vi "SAOMM-FalconFixer.vi"(0 "PRAMMS VRN":refnum<visa-resource-name>="COM4", 1 "ROIYOffset":u16, 2 "ROIXOffset":u16, 3 "Binning":u16(ring) items=["1 x 1"=1, "2 x 2"=2, "4 x 4"=4, "5 x 5"=5], 7 "Signature":u32, 11 "PRAMMS Error":errorcluster, 12 "ROIWidth":u16, 13 "ROIHeight":u16) -> ()   [LabVIEW 2011]
uses:
  Polymorphics/Num2littleEndian(U16).vi
panel:
  out "appended array 2":bool[](array[boolean])
  out "DumpArray1":string[](array[string])
  out "appended array":bool[](array[boolean])
  out "Boolean":bool
  out "DumpArray2":string[](array[string])
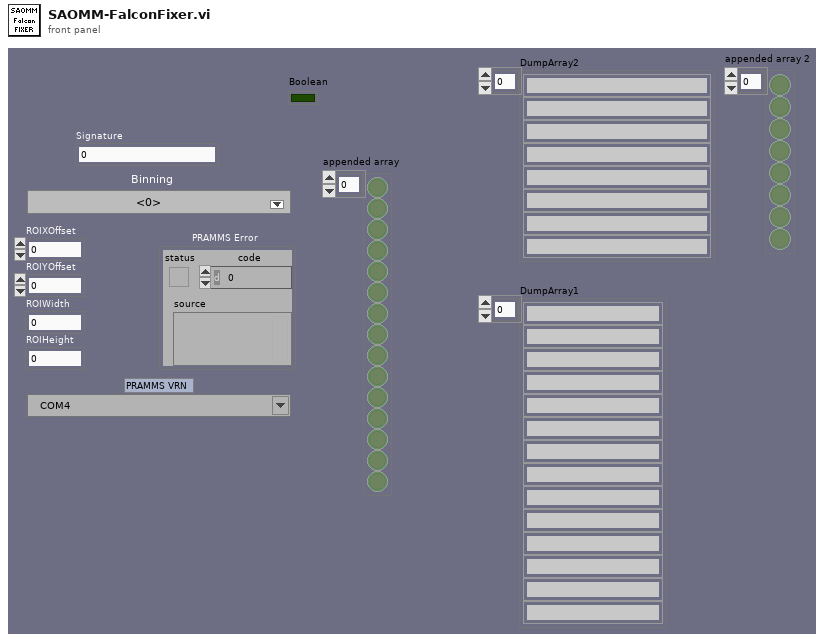
[diagram p1: front panel]
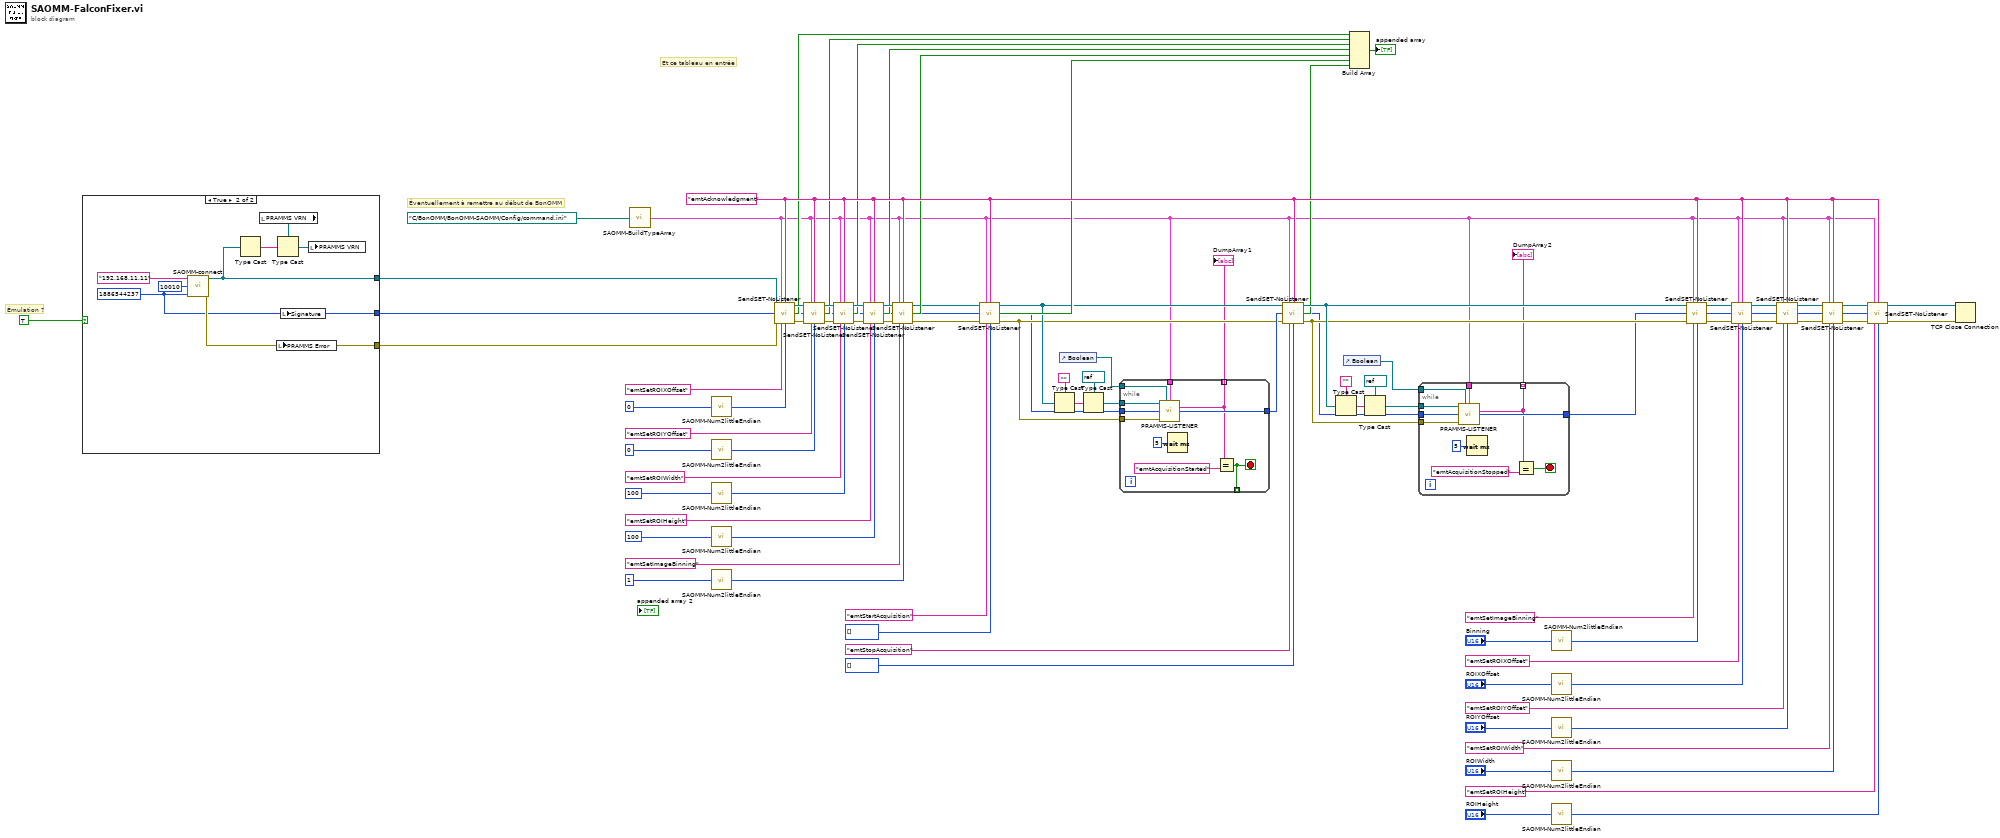
[diagram p0: block diagram]
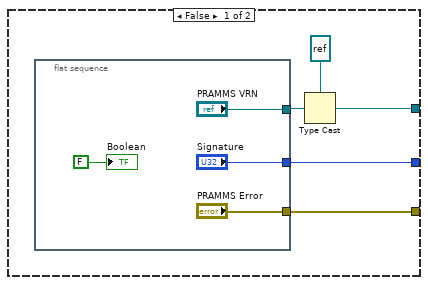
[diagram p2: hidden frame]
diagram:
  w48 = "emtAcknowledgment" ("ExpectedAnswer")
  # "Émulation ?"
  # "Et ce tableau en entrée"
  # "Éventuellement à remettre au début de BonOMM"
  n1 = case shown="True" TRUE {
    tunnel: [w92 w97] -> w69
    tunnel: [w89 w102] -> w50
    tunnel: [w88 w101] -> w3
    frame False {
      n2 = flat-sequence {
        tunnel: ["PRAMMS VRN"] -> w90
        tunnel: ["PRAMMS Error"] -> w89
        tunnel: ["Signature"] -> w88
        frame #0 {
          "Boolean" <- FALSE
        }
      }
      n3 = Type Cast(type=refnum<k5> refnum ("connection ID"), x=w90) -> (*(type *) &x=w92:refnum<k5>)
    }
    frame True {
      w101 = u32 1886544237 ("Signature")
      n4 = call "SAOMM-connect.vi"("IP"="192.168.11.11", "Port"=u16 10010, "Signature"=w101) -> ("connection ID"=w97:refnum<k5>, "Error OUT"=w102:errorcluster)  [unwired: 8 in, 3 out]
      n5 = Type Cast(x=w97) -> (*(type *) &x=w98:string)  [unwired: 1 in]
      n6 = local read "PRAMMS VRN"() -> (w100:refnum<visa-resource-name>)
      n7 = local write "PRAMMS Error"(w102) -> ()
      n8 = Type Cast(type=w100, x=w98) -> (*(type *) &x=w99:refnum<visa-resource-name>)
      n9 = local write "Signature"(w101) -> ()
      n10 = local write "PRAMMS VRN"(w99) -> ()
    }
  }
  n11 = call "SAOMM-BuildTypeArray.vi"("command.ini"=path "C:/BonOMM/BonOMM-SAOMM/Config/command.ini") -> ("CommandArray"=w9:cluster{string[], u32[]})  [unwired: 14 in]
  n12 = call-poly "SAOMM-Num2littleEndian.vi"("Number"=u16 0) -> ("LiitleEndianedData"=w63:u8[])  [unwired: 14 in]
  n13 = call-poly "SAOMM-Num2littleEndian.vi"("Number"=u16 0) -> ("LiitleEndianedData"=w62:u8[])  [unwired: 14 in]
  n14 = call-poly "SAOMM-Num2littleEndian.vi"("Number"=u16 100) -> ("LiitleEndianedData"=w61:u8[])  [unwired: 14 in]
  n15 = call-poly "SAOMM-Num2littleEndian.vi"("Number"=u16 100) -> ("LiitleEndianedData"=w60:u8[])  [unwired: 14 in]
  n16 = call-poly "SAOMM-Num2littleEndian.vi"("Number"=u16 1) -> ("LiitleEndianedData"=w56:u8[])  [unwired: 14 in]
  n17 = call "SendSET-NoListener.vi"("connection ID"=w69, "CommandArray"=w9, "ExpectedAnswer"=w48, "Signature"=w3, "Error IN"=w50, "Active SET"="emtSetROIXOffset", "Value (little endianed byte array)"=w63) -> ("connection ID (dup)"=w82:refnum<k5>, "Succes"=w25:bool, "Error OUT"=w68:errorcluster)  [unwired: 6 in]
  n18 = call "SendSET-NoListener.vi"("connection ID"=w82, "CommandArray"=w9, "ExpectedAnswer"=w48, "Signature"=w3, "Error IN"=w68, "Active SET"="emtSetROIYOffset", "Value (little endianed byte array)"=w62) -> ("connection ID (dup)"=w81:refnum<k5>, "Succes"=w24:bool, "Error OUT"=w73:errorcluster)  [unwired: 6 in]
  n19 = call "SendSET-NoListener.vi"("connection ID"=w81, "CommandArray"=w9, "ExpectedAnswer"=w48, "Signature"=w3, "Error IN"=w73, "Active SET"="emtSetROIWidth", "Value (little endianed byte array)"=w61) -> ("connection ID (dup)"=w80:refnum<k5>, "Succes"=w23:bool, "Error OUT"=w70:errorcluster)  [unwired: 6 in]
  n20 = call "SendSET-NoListener.vi"("connection ID"=w80, "CommandArray"=w9, "ExpectedAnswer"=w48, "Signature"=w3, "Error IN"=w70, "Active SET"="emtSetROIHeight", "Value (little endianed byte array)"=w60) -> ("connection ID (dup)"=w58:refnum<k5>, "Succes"=w22:bool, "Error OUT"=w57:errorcluster)  [unwired: 6 in]
  n21 = call "SendSET-NoListener.vi"("connection ID"=w58, "CommandArray"=w9, "ExpectedAnswer"=w48, "Signature"=w3, "Error IN"=w57, "Active SET"="emtSetImageBinning", "Value (little endianed byte array)"=w56) -> ("connection ID (dup)"=w4:refnum<k5>, "Succes"=w18:bool, "Error OUT"=w2:errorcluster)  [unwired: 6 in]
  n22 = call "SendSET-NoListener.vi"("connection ID"=w4, "CommandArray"=w9, "ExpectedAnswer"=w48, "Signature"=w3, "Error IN"=w2, "Active SET"="emtStartAcquisition", "Value (little endianed byte array)"=u8[] []) -> ("connection ID (dup)"=w14:refnum<k5>, "Succes"=w21:bool, "Error OUT"=w11:errorcluster)  [unwired: 6 in]
  n23 = Type Cast(type="", x=w14) -> (*(type *) &x=w17:string)
  n24 = control-ref of="Boolean"() -> (w10:refnum<vi>)
  n25 = Type Cast(type=refnum<visa-resource-name> refnum ("PRAMMS VRN"), x=w17) -> (*(type *) &x=w13:refnum<visa-resource-name>)
  n26 = while {
    tunnel: w13 -> [w113]
    tunnel: w11 -> [w112]
    tunnel: w3 -> [w110]
    tunnel: [w110] -> w12
    tunnel: [w108] -> w8 mode=indexing
    tunnel: w10 -> [w107]
    tunnel: w9 -> [w106]
    tunnel: [w105] -> _ mode=indexing
    stop <- w105 stop-if-true
    n27 = call "PRAMMS-LISTENER.vi"("PRAMMS-COMM IN"=w113, "Bool Refnum"=w107, "MessageTypeArray"=w106, "Signature"=w110, "Error IN"=w112) -> ("Type"=w108:string)  [unwired: 5 in, 5 out]
    n28 = Wait (ms)(milliseconds to wait=u32 5) -> ()  [unwired: 1 out]
    n29 = Equal?(x=w108, y="emtAcquisitionStarted") -> (x = y?=w105:bool)
  }
  "DumpArray1" <- w8
  n30 = call "SendSET-NoListener.vi"("connection ID"=w14, "CommandArray"=w9, "ExpectedAnswer"=w48, "Signature"=w12, "Error IN"=w11, "Active SET"="emtStopAcquisition", "Value (little endianed byte array)"=u8[] []) -> ("connection ID (dup)"=w34:refnum<k5>, "Succes"=w20:bool, "Error OUT"=w33:errorcluster)  [unwired: 6 in]
  n31 = Type Cast(type="", x=w34) -> (*(type *) &x=w36:string)
  n32 = control-ref of="Boolean"() -> (w30:refnum<vi>)
  n33 = Build Array(w25, w24, w23, w22, w18, w21, w20) -> (→"appended array":bool[])
  n34 = Type Cast(type=refnum<visa-resource-name> refnum ("PRAMMS VRN"), x=w36) -> (*(type *) &x=w35:refnum<visa-resource-name>)
  n35 = while {
    tunnel: w35 -> [w122]
    tunnel: w33 -> [w121]
    tunnel: w12 -> [w118]
    tunnel: [w118] -> w32
    tunnel: [w116] -> w31 mode=indexing
    tunnel: w30 -> [w115]
    tunnel: w9 -> [w114]
    stop <- w119 stop-if-true
    n36 = call "PRAMMS-LISTENER.vi"("PRAMMS-COMM IN"=w122, "Bool Refnum"=w115, "MessageTypeArray"=w114, "Signature"=w118, "Error IN"=w121) -> ("Type"=w116:string)  [unwired: 5 in, 5 out]
    n37 = Wait (ms)(milliseconds to wait=u32 5) -> ()  [unwired: 1 out]
    n38 = Equal?(x=w116, y="emtAcquisitionStopped") -> (x = y?=w119:bool)
  }
  "DumpArray2" <- w31
  n39 = call-poly "SAOMM-Num2littleEndian.vi"("Number"="Binning") -> ("LiitleEndianedData"=w83:u8[])  [unwired: 14 in]
  n40 = call-poly "SAOMM-Num2littleEndian.vi"("Number"="ROIXOffset") -> ("LiitleEndianedData"=w84:u8[])  [unwired: 14 in]
  n41 = call-poly "SAOMM-Num2littleEndian.vi"("Number"="ROIYOffset") -> ("LiitleEndianedData"=w85:u8[])  [unwired: 14 in]
  n42 = call-poly "SAOMM-Num2littleEndian.vi"("Number"="ROIWidth") -> ("LiitleEndianedData"=w86:u8[])  [unwired: 14 in]
  n43 = call-poly "SAOMM-Num2littleEndian.vi"("Number"="ROIHeight") -> ("LiitleEndianedData"=w87:u8[])  [unwired: 14 in]
  n44 = call "SendSET-NoListener.vi"("connection ID"=w34, "CommandArray"=w9, "ExpectedAnswer"=w48, "Signature"=w32, "Error IN"=w33, "Active SET"="emtSetImageBinning", "Value (little endianed byte array)"=w83) -> ("connection ID (dup)"=w79:refnum<k5>, "Error OUT"=w71:errorcluster)  [unwired: 6 in, 1 out]
  n45 = call "SendSET-NoListener.vi"("connection ID"=w79, "CommandArray"=w9, "ExpectedAnswer"=w48, "Signature"=w32, "Error IN"=w71, "Active SET"="emtSetROIXOffset", "Value (little endianed byte array)"=w84) -> ("connection ID (dup)"=w78:refnum<k5>, "Error OUT"=w74:errorcluster)  [unwired: 6 in, 1 out]
  n46 = call "SendSET-NoListener.vi"("connection ID"=w78, "CommandArray"=w9, "ExpectedAnswer"=w48, "Signature"=w32, "Error IN"=w74, "Active SET"="emtSetROIYOffset", "Value (little endianed byte array)"=w85) -> ("connection ID (dup)"=w77:refnum<k5>, "Error OUT"=w72:errorcluster)  [unwired: 6 in, 1 out]
  n47 = call "SendSET-NoListener.vi"("connection ID"=w77, "CommandArray"=w9, "ExpectedAnswer"=w48, "Signature"=w32, "Error IN"=w72, "Active SET"="emtSetROIWidth", "Value (little endianed byte array)"=w86) -> ("connection ID (dup)"=w76:refnum<k5>, "Error OUT"=w75:errorcluster)  [unwired: 6 in, 1 out]
  n48 = call "SendSET-NoListener.vi"("connection ID"=w76, "CommandArray"=w9, "ExpectedAnswer"=w48, "Signature"=w32, "Error IN"=w75, "Active SET"="emtSetROIHeight", "Value (little endianed byte array)"=w87) -> ("connection ID (dup)"=w6:refnum<k5>, "Error OUT"=w5:errorcluster)  [unwired: 6 in, 1 out]
  n49 = TCP Close Connection(connection ID=w6, error in (no error)=w5) -> ()  [unwired: 1 in, 2 out]
